vi "SET_PRODUCT_STATUS.vi"() -> ()   [LabVIEW 2020]
panel:
  in  "取消":bool
  in  "确定":bool
  in  "设置状态":enum16{"", "OK", "NG"}(ring)
  out "当前状态":string
  in  "设备名称":u16(ring) caption="Enum 3" items=["", "芯轴分总成磨合台", "上管柱组件装配", "上管柱上转向轴合成", "滑移力检测", "芯轴分总成NVH", "上转向轴组件装配", "上下管柱总成装配", "滑移力复检", "最终性能试验台", "传感器对中台", "电机装配", "中间轴装配", "GP12（340）", "ECU装配", "激光打标机"]
  in  "追溯码":string
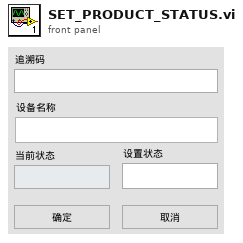
[diagram p1: front panel]
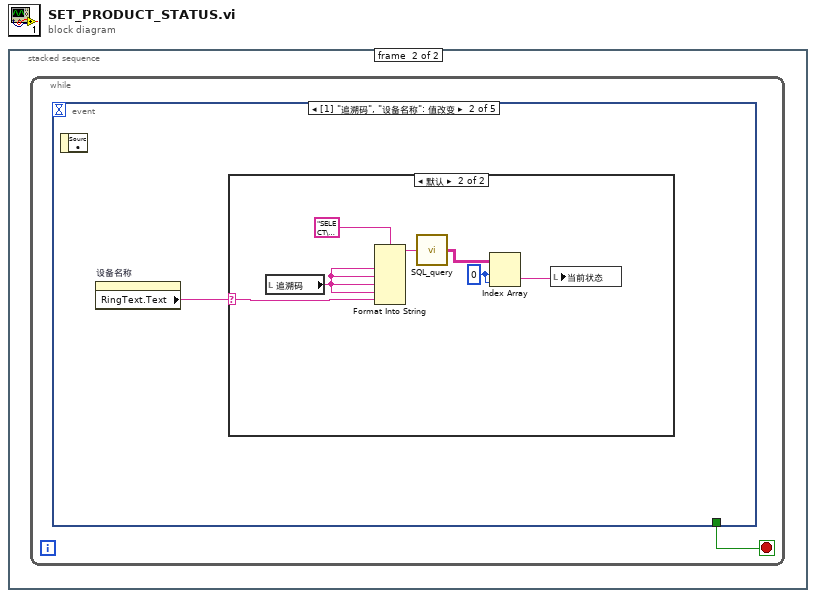
[diagram p0: block diagram]
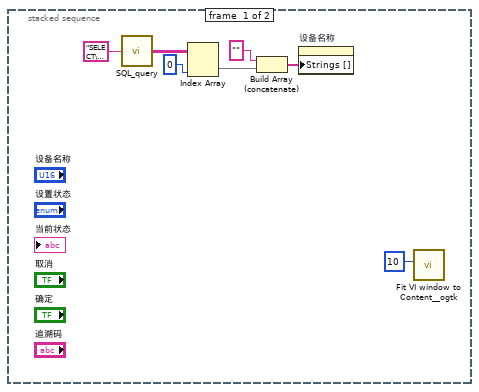
[diagram p2: hidden frame]
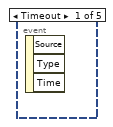
[diagram p3: hidden frame]
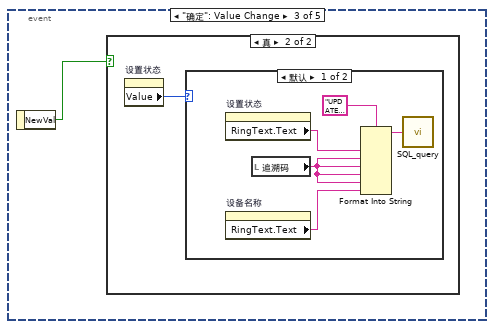
[diagram p5: hidden frame]
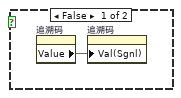
[diagram p6: hidden frame]
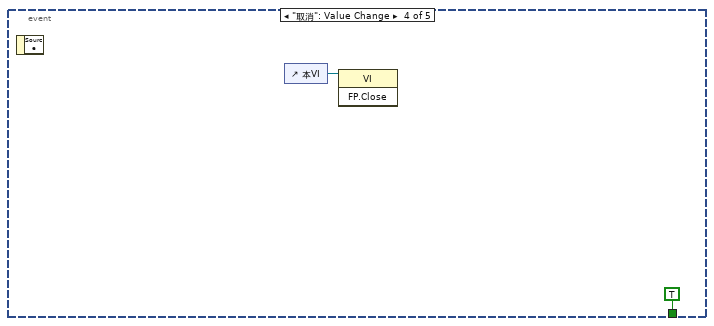
[diagram p8: hidden frame]
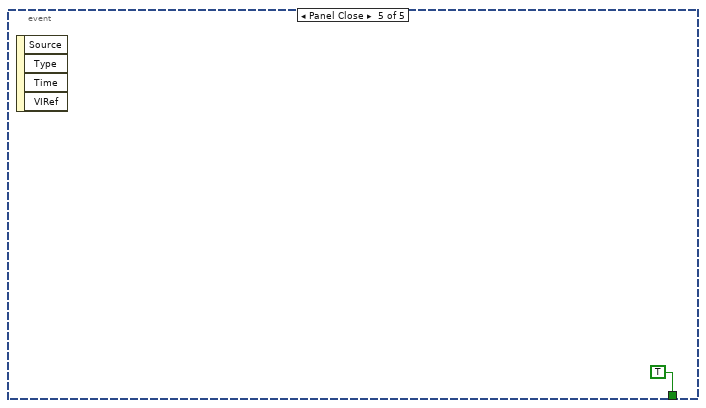
[diagram p9: hidden frame]
diagram:
  n1 = stacked-sequence {
    frame #0 {
      n2 = call "SQL_query.vi"("SQL query"="SELECT\ndbo.Device.DEVICE_NAME\n\nFROM\ndbo.Device\n") -> ("data"=w6:string[][])  [unwired: 3 in, 1 out]
      n3 = Index Array(array=w6, index (col)=0 ("禁用的索引 (列)")) -> (element=w5:string[])  [unwired: 1 in]
      n4 = Build Array (concatenate)("", w5) -> (w2:string[])
      n5 = property on="设备名称" class="Ring (严格)"("Strings []"=w2) -> ()  [unwired: 2 in, 2 out]
      n6 = call <userlib>:"Fit VI window to Content__ogtk.vi"("border spacing (2 px)"=10) -> ()  [unwired: 5 in, 2 out]
    }
    frame #1 {
      n7 = while {
        stop <- w8 stop-if-true
        n8 = event shown="[1] \"追溯码\", \"设备名称\": 值改变" {
          selector: _ -> [_ _ _ _ _]
          dyn-events: _ -> [_ _ _ _ _]
          timeout: _ -> [_ _ _ _ _]
          tunnel: [_ _ _ TRUE TRUE] -> w8
          event Timeout {
            n9 = event-data() -> ()  [unwired: 1 in, 3 out]
          }
          event "追溯码", "设备名称": Value Change {
            n10 = event-data() -> ()  [unwired: 1 in, 1 out]
            n11 = property on="设备名称" class="Ring (严格)"() -> ("RingText.Text"=w9:string)  [unwired: 2 in, 2 out]
            n12 = case shown="默认" w9 {
              selector: w9 -> [_ w14]
              frame "" {
              }
              frame Default {
                w12 = 0 ("索引 (行)")
                n13 = local read "追溯码"() -> (w16:string)
                n14 = Format Into String(format string="SELECT\n[dbo].[Result].[RESULT_VALUE] \nFROM\ndbo.Result\nINNER JOIN dbo.Code ON dbo.Result.CODE_ID = dbo.Code.CODE_ID\nINNER JOIN dbo.Device ON dbo.Result.DEVICE_ID = dbo.Device.DEVICE_ID\nWHERE\n(dbo.Code.CODE_MAIN = '%s' OR\ndbo.Code.CODE_SENSOR = '%s' OR\ndbo.Code.CODE_MOTOR = '%s' OR\ndbo.Code.CODE_ECU = '%s' ) AND\ndbo.Device.DEVICE_NAME = '%s'\n" ("格式字符串"), w16, w16, w16, w16, w14) -> (resulting string=w15:string)  [unwired: 2 in, 1 out]
                n15 = call "SQL_query.vi"("SQL query"=w15) -> ("data"=w13:string[][])  [unwired: 3 in, 1 out]
                n16 = Index Array(array=w13, index (row)=w12, index (col)=w12) -> (element=w11:string)
                n17 = local write "当前状态"(w11) -> ()
              }
            }
          }
          event "确定": Value Change {
            n18 = event-data() -> ("NewVal"=w17:bool)  [unwired: 1 in]
            n19 = case shown="真" w17 {
              frame False {
                n20 = property on="追溯码" class="Str"() -> ("Value"=w18:string)  [unwired: 2 in, 2 out]
                n21 = property on="追溯码" class="Str"("Val(Sgnl)"=w18) -> ()  [unwired: 2 in, 2 out]
              }
              frame True {
                n22 = property on="设置状态" class="Enum (严格)"() -> ("Value"=w19:enum16{"", "OK", "NG"})  [unwired: 2 in, 2 out]
                n23 = case shown="默认" w19 {
                  frame Default {
                    n24 = property on="设置状态" class="Enum (严格)"() -> ("RingText.Text"=w21:string)  [unwired: 2 in, 2 out]
                    n25 = property on="设备名称" class="Ring (严格)"() -> ("RingText.Text"=w23:string)  [unwired: 2 in, 2 out]
                    n26 = local read "追溯码"() -> (w24:string)
                    n27 = Format Into String(format string="UPDATE \n[dbo].[Result] \nSET \n[RESULT_VALUE] = N'%s'\nFROM\ndbo.Result\nINNER JOIN dbo.Code ON dbo.Result.CODE_ID = dbo.Code.CODE_ID\nINNER JOIN dbo.Device ON dbo.Result.DEVICE_ID = dbo.Device.DEVICE_ID\nWHERE\n(dbo.Code.CODE_MAIN = '%s' OR\ndbo.Code.CODE_SENSOR = '%s' OR\ndbo.Code.CODE_MOTOR = '%s' OR\ndbo.Code.CODE_ECU = '%s' ) AND\ndbo.Device.DEVICE_NAME = '%s'\n" ("格式字符串"), w21, w24, w24, w24, w24, w23) -> (resulting string=w22:string)  [unwired: 2 in, 1 out]
                    n28 = call "SQL_query.vi"("SQL query"=w22) -> ()  [unwired: 3 in, 2 out]
                  }
                  frame "" {
                  }
                }
              }
            }
          }
          event "取消": Value Change {
            n29 = event-data() -> ()  [unwired: 1 in, 1 out]
            n30 = control-ref of="本VI"() -> (w25:refnum<vi>)
            n31 = invoke class="VI" method="FP.Close"(reference=w25) -> ()  [unwired: 2 in, 3 out]
          }
          event Panel Close {
            n32 = event-data() -> ()  [unwired: 1 in, 4 out]
          }
        }
      }
    }
  }
